vi "3Act Helper - ReadPWMFindEdge.vi"(8 "Remote Control DIO Error":errorcluster, 10 "For loop cycles (100)":i32=100, 11 "Remote Control DIO Reference":T1) -> (0 "error out":errorcluster, 3 "Averaged digital line values":dbl[](array[numeric]))   [LabVIEW 2013]
doc: "Reads in a digital line for a set number of cycles, then calculates the average value over those cycles. This is meant to give us a rough estimation for a PWM value. It's unclear whether the MyRI Odigital sampling will be too slow or not to get steady data for the PWM value.\n\nEric Schneider, May 2014"
uses:
  <vilib>/myRIO/Instrument Drivers/Onboard IO/DIO/typedefs/DIO Reference.ctl
  <vilib>/myRIO/Common/Instrument Driver Framework/Utilities/typedefs/myRIO Generic Hardware Reference.ctl
  <vilib>/myRIO/Common/Instrument Driver Framework/Utilities/typedefs/Hardware Version Enum.ctl
  <vilib>/myRIO/Common/Instrument Driver Framework/Utilities/typedefs/myRIO v1.0 Reference.ctl
  <vilib>/myRIO/Common/Instrument Driver Framework/Utilities/typedefs/Generic FPGA Reference.ctl
  <vilib>/myRIO/Common/Instrument Driver Framework/myRIO v1.0/DIO/typedefs/DIO Channels List.ctl
  <vilib>/myRIO/Common/Instrument Driver Framework/myRIO v1.0/DIO/typedefs/DIO Channels Enum.ctl
  <vilib>/Utility/error.llb/Error Cluster From Error Code.vi
  <vilib>/myRIO/Common/Instrument Driver Framework/myRIO v1.0/DIO/vis/myRIO v1.0 Read DIO.vi
  <vilib>/myRIO/Instrument Drivers/Onboard IO/DIO/DIO.lvlib
panel:
  out "Values":bool[](array[boolean])
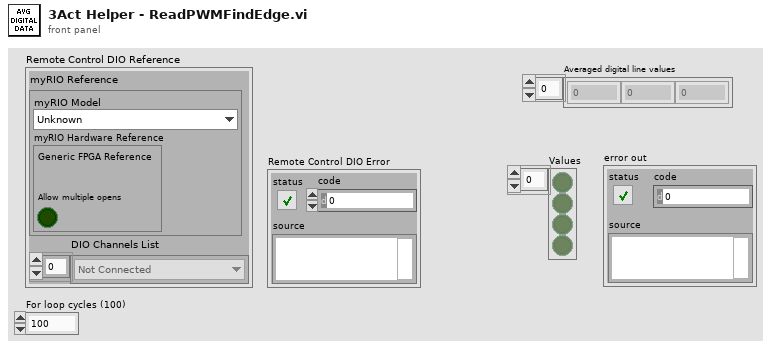
[diagram p1: front panel]
types:
  T1 = typedef "DIO.lvlib/DIO Reference.ctl" = cluster{"myRIO Reference":T2, "DIO Channels List":T6}
  T2 = typedef "myRIO Generic Hardware Reference.ctl" = cluster{"myRIO Model":T3, "myRIO Hardware Reference":T4}
  T3 = typedef "Hardware Version Enum.ctl" = enum16{"Unknown", "myRIO-1900", "myRIO-1950"}
  T4 = typedef "myRIO v1.0 Reference.ctl" = cluster{"Generic FPGA Reference":T5, "Allow multiple opens":bool}
  T5 = typedef "Generic FPGA Reference.ctl" = refnum<k20>
  T6 = typedef "DIO Channels List.ctl" = T7[]
  T7 = typedef "DIO Channels Enum.ctl" = enum16{"Not Connected", "C/DIO0", "C/DIO1", "C/DIO2", "C/DIO3", "C/DIO4", "C/DIO5", "C/DIO6", "C/DIO7", "A/DIO0", "A/DIO1", "A/DIO2", "A/DIO3", "A/DIO4", "A/DIO5", "A/DIO6", "A/DIO7", "A/DIO8", "A/DIO9", "A/DIO10", "A/DIO11", "A/DIO12", "A/DIO13", "A/DIO14", "A/DIO15", "B/DIO0", "B/DIO1", "B/DIO2", "B/DIO3", "B/DIO4", "B/DIO5", "B/DIO6", "B/DIO7", "B/DIO8", "B/DIO9", "B/DIO10", "B/DIO11", "B/DIO12", "B/DIO13", "B/DIO14", "B/DIO15", "LED0", "LED1", "LED2", "LED3", "Button0"}
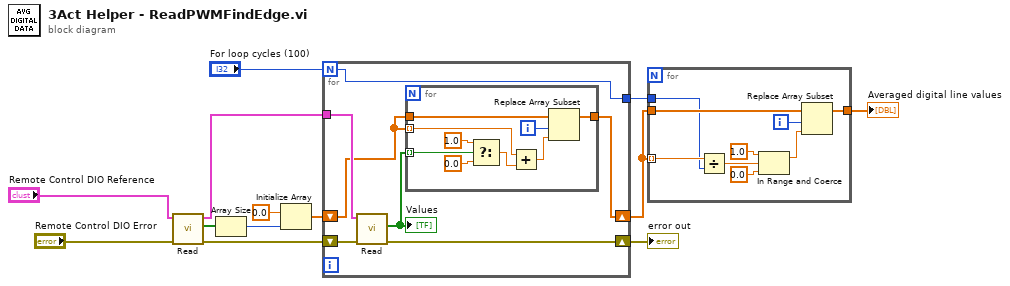
[diagram p0: block diagram]
diagram:
  n1 = call <vilib>:"Read.vi"("error in (no error)"="Remote Control DIO Error", "DIO Ref In"="Remote Control DIO Reference") -> ("error out"=w10:errorcluster, "Values"=w5:bool[], "DIO Ref Out"=w6:T1)  [unwired: 7 in]
  n2 = Array Size(array=w5) -> (size(s)=w9:i32)
  n3 = Initialize Array(0.0 ("element"), w9) -> (w7:dbl[])
  n4 = for {
    N: "For loop cycles (100)" -> [w16]
    tunnel: w6 -> [w20]
    shift-right: [w17] -> w4
    shift-left: w7 -> [w15]
    tunnel: [w16] -> w1
    shift-right: [w14] -> w2
    shift-left: w10 -> [w19]
    n5 = call <vilib>:"Read.vi"("error in (no error)"=w19, "DIO Ref In"=w20) -> ("error out"=w14:errorcluster, "Values"=w18:bool[])  [unwired: 7 in, 1 out]
    "Values" <- w18
    n6 = for {
      tunnel: w18 -> [w29] mode=indexing
      tunnel: w15 -> [w21] mode=indexing
      tunnel: [w23] -> w17
      tunnel: w15 -> [w22]
      i -> [w26]
      n7 = Select(t=1.0, s=w29, f=0.0) -> (s? t:f=w25:dbl)
      n8 = Add(x=w21, y=w25) -> (x+y=w24:dbl)
      n9 = Replace Array Subset(array=w22, new element=w24, index=w26) -> (w23:dbl[])
    }
  }
  "error out" <- w2
  n10 = for {
    tunnel: w4 -> [w36]
    tunnel: w4 -> [w38] mode=indexing
    tunnel: [w35] -> w3
    tunnel: w1 -> [w34]
    i -> [w37]
    n11 = Divide(x=w38, y=w34) -> (x/y=w33:dbl)
    n12 = In Range and Coerce(upper limit=1.0, x=w33, lower limit=0.0) -> (coerced(x)=w32:dbl)  [unwired: 1 out]
    n13 = Replace Array Subset(array=w36, new element=w32, index=w37) -> (w35:dbl[])
  }
  "Averaged digital line values" <- w3
